vi "Hysteresis-NormalizedArray.vi"(11 "Array in":dbl[](array[numeric])) -> (3 "Array out":dbl[](array[numeric]))   [LabVIEW 2016]
uses:
  <vilib>/Analysis/baseanly.llb/Mean (DBL).vi
  <vilib>/Analysis/NI_AALBase.lvlib
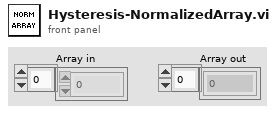
[diagram p1: front panel]
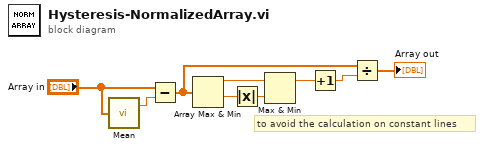
[diagram p0: block diagram]
diagram:
  # "to avoid the calculation on constant lines"
  n1 = call-poly <vilib>:"Mean.vi"("X"="Array in") -> ("mean"=w1:dbl)  [unwired: 1 out]
  n2 = Subtract(x="Array in", y=w1) -> (x-y=w8:dbl[])
  n3 = Array Max & Min(array=w8) -> (max value=w5:dbl, min value=w3:dbl)  [unwired: 2 out]
  n4 = Absolute Value(x=w3) -> (abs(x)=w4:dbl)
  n5 = Max & Min(x=w5, y=w4) -> (max(x,y)=w6:dbl)  [unwired: 1 out]
  n6 = Increment(x=w6) -> (x+1=w7:dbl)
  n7 = Divide(x=w8, y=w7) -> (x/y=→"Array out":dbl[])
